vi "Initialize Main to Subpanel Command.vi"(8 "error in (no error)":errorcluster) -> (0 "error out":errorcluster, 2 "main to subpanel command event reg":T2, 3 "main to subpanel command event":T1)   [LabVIEW 2017, in "NI_Robotics_Configure Steering Frame.lvlib"]
uses:
  <vilib>/robotics/Dialog/Configure Steering Frame/NI_Robotics_Configure Steering Frame.lvlib
  <vilib>/robotics/Dialog/Configure Steering Frame/Main to Subpanel Command Event Reg.ctl
  <vilib>/robotics/Dialog/Configure Steering Frame/Main to Subpanel Command.ctl
  <vilib>/robotics/Steering/Steering Frame/NI_Robotics_Steering Frame.lvclass
  <vilib>/robotics/Dialog/Configure Steering Frame/Main to Subpanel Command Event.ctl
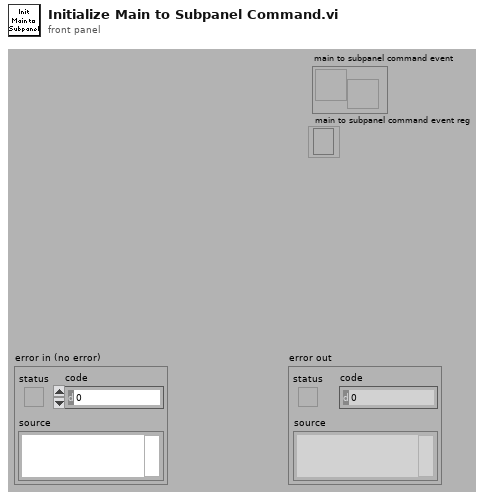
[diagram p1: front panel]
types:
  T1 = typedef "NI_Robotics_Configure Steering Frame.lvlib/Main to Subpanel Command Event.ctl" = refnum<user-event>
  T2 = typedef "NI_Robotics_Configure Steering Frame.lvlib/Main to Subpanel Command Event Reg.ctl" = refnum<event-registration>
  T3 = typedef "NI_Robotics_Configure Steering Frame.lvlib/Main to Subpanel Command.ctl" = cluster{"command":string, "steering frame reference":refnum<data-value>, "active wheel indexes":i32[]}
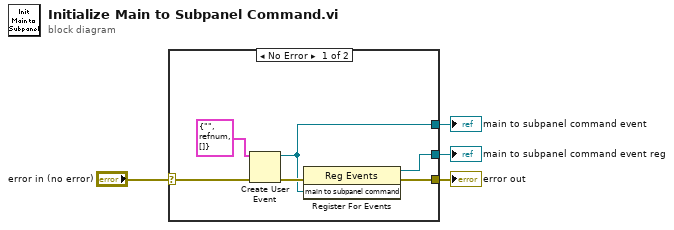
[diagram p0: block diagram]
diagram:
  n1 = case shown="No Error" "error in (no error)" {
    selector: "error in (no error)" -> [w9 w11]
    tunnel: [w7 _] -> w3
    tunnel: [w6 _] -> w1
    tunnel: [w5 w11] -> w2
    frame No Error {
      n2 = Create User Event(user event datatype=T3 {"command"="", "steering frame reference"=refnum, "active wheel indexes"=[]} ("main to subpanel command"), error in=w9) -> (user event=w7:refnum<user-event>, error out=w8:errorcluster)
      n3 = register-events(error in=w8, w7) -> (reference out=w6:refnum<event-registration>, error out=w5:errorcluster)  [unwired: 1 in]
    }
    frame Error {
    }
  }
  "error out" <- w2
  "main to subpanel command event reg" <- w1
  "main to subpanel command event" <- w3
